vi "4.6.vi"() -> ()   [LabVIEW 2019]
uses:
  <vilib>/imath/engines/lvmath2/RunTimeEngine/RangeToken/NIMS_Range.vi
  <instcachedir>/0/NIMS_Range_0856D726B6B24596B614846B21C682A9.lvgen/NIMS_Range_0856D726B6B24596B614846B21C682A9_000.vi
  <vilib>/imathl/engines/lvmath/Functions/Error Handling/Create Error.vi
  <vilib>/imath/engines/lvmath2/RunTimeEngine/ArithmeticOperatorToken/NIMS_ArithmeticOperator_multmx.vi
  <instcachedir>/0/NIMS_ArithmeticOperator_multmx_99144D996F2B45CCBE745A128A95DE55.lvgen/NIMS_ArithmeticOperator_multmx_99144D996F2B45CCBE745A128A95DE55_004.vi
  <vilib>/imath/engines/lvmath2/RunTimeEngine/ArithmeticOperatorToken/NIMS_ArithmeticOperator_powermx(M,M).vi
  <vilib>/imath/engines/lvmath2/RunTimeEngine/ArithmeticOperatorToken/NIMS_ArithmeticOperator_plus.vi
  <instcachedir>/0/NIMS_ArithmeticOperator_plus_A857F7369B7D4E138264023AAAB8243E.lvgen/NIMS_ArithmeticOperator_plus_A857F7369B7D4E138264023AAAB8243E_011.vi
  <instcachedir>/0/NIMS_ArithmeticOperator_plus_A857F7369B7D4E138264023AAAB8243E.lvgen/NIMS_ArithmeticOperator_plus_A857F7369B7D4E138264023AAAB8243E_010.vi
  <vilib>/imath/engines/lvmath2/RunTimeEngine/NodeEndStatement/NIMS_NodeEndStatement_Get Scalar.vi
  <instcachedir>/0/NIMS_NodeEndStatement_Get Scalar_0303A3DA16E64F8AA7C32B7099803384.lvgen/NIMS_NodeEndStatement_Get Scalar_0303A3DA16E64F8AA7C32B7099803384_000.vi
  <vilib>/imath/engines/lvmath2/RunTimeEngine/NodeEndStatement/NIMS_NodeEndStatement_Output.vi
  <instcachedir>/0/NIMS_NodeEndStatement_Output_53EC0D466D134D7ABD903AC30B43404B.lvgen/NIMS_NodeEndStatement_Output_53EC0D466D134D7ABD903AC30B43404B_001.vi
  <vilib>/imath/engines/lvmath2/RunTimeEngine/ErrorHandling/NIMS_Finalize Error.vi
panel:
  out "R":dbl
  in  "h":dbl
  in  "v":dbl
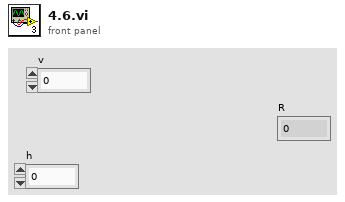
[diagram p1: front panel]
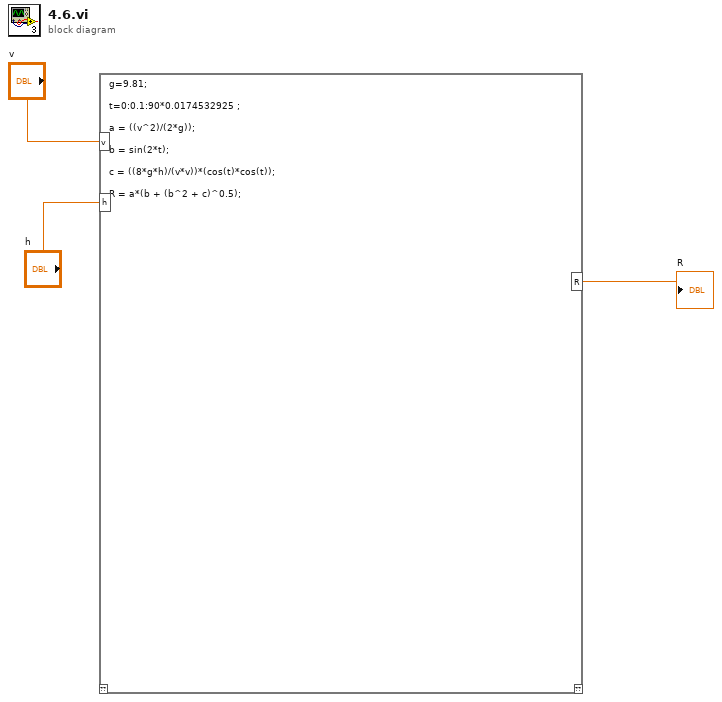
[diagram p0: block diagram]
diagram:
  n1 = mathscript code="g=9.81;\n\nt=0:0.1:90*0.0174532925 ;\n\na = ((v^2)/(2*g));\n\nb = sin(2*t);\n\nc = ((8*g*h)/(v*v))*(cos(t)*cos(t));\n\nR = a*(b + (b^2 + c)^0.5);"("v"="v", "h"="h") -> ("R"=→"R":dbl)  [unwired: 1 in, 1 out]
